vi "Set BUZZ.vi"(10 "Inetensity":dbl, 11 "BUZZ Select":T1) -> (3 "Controller BUZZ":T2)   [LabVIEW 2020, in "GameController_SEN.lvlib"]
uses:
  GameController_SEN.lvlib
  Shared Code/TypeDefs/Cluster_Controller Buzz.ctl
  Shared Code/TypeDefs/ENUM_Controller Buzz Select.ctl
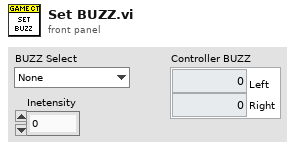
[diagram p1: front panel]
types:
  T1 = typedef "ENUM_Controller Buzz Select.ctl" = enum16{"None", "Timed Full ON", "Set Intensity", ".5 Sec Cycle Count"}
  T2 = typedef "Cluster_Controller Buzz.ctl" = cluster{"Left":dbl, "Right":dbl}
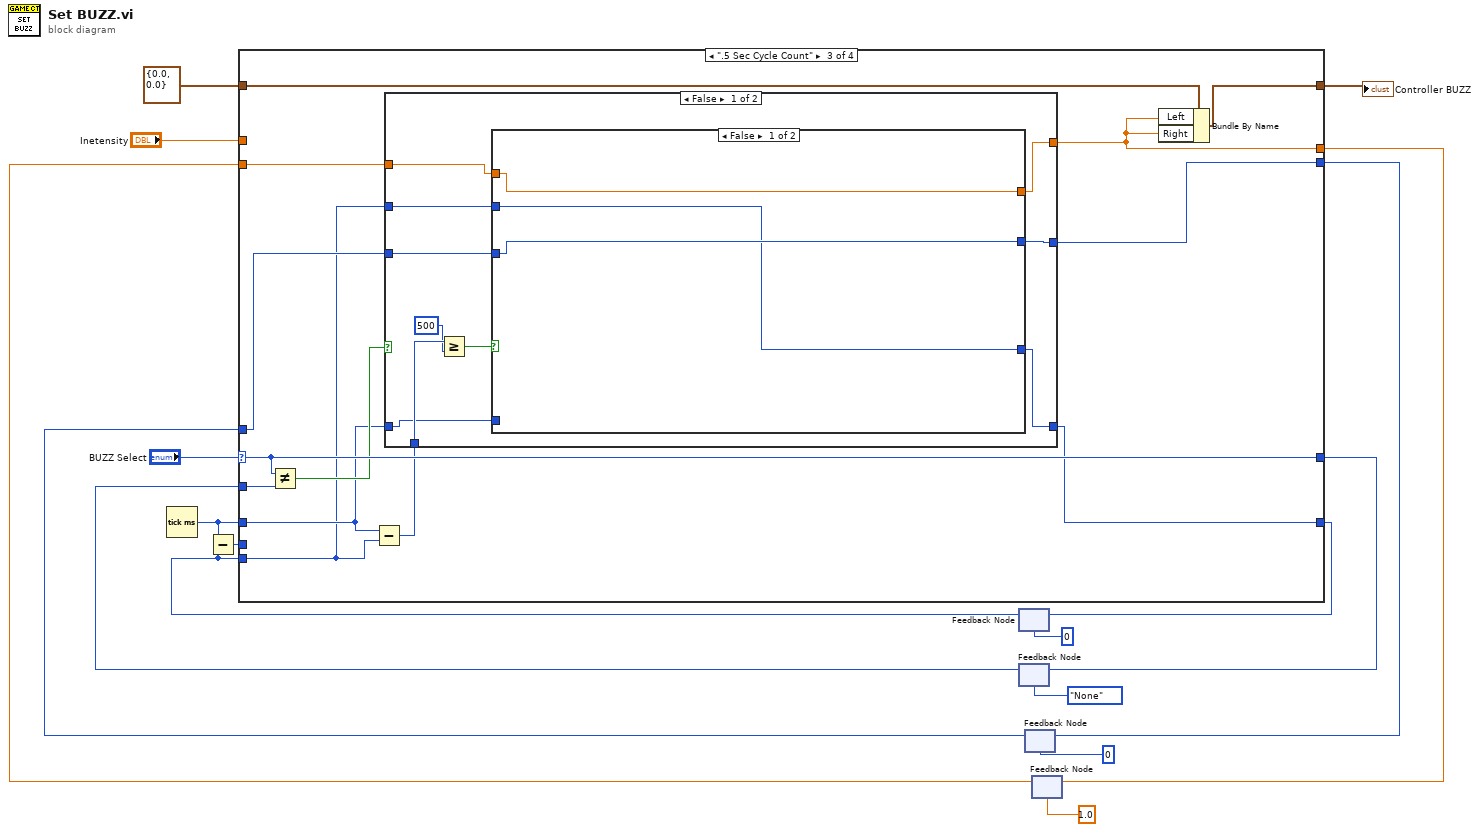
[diagram p0: block diagram]
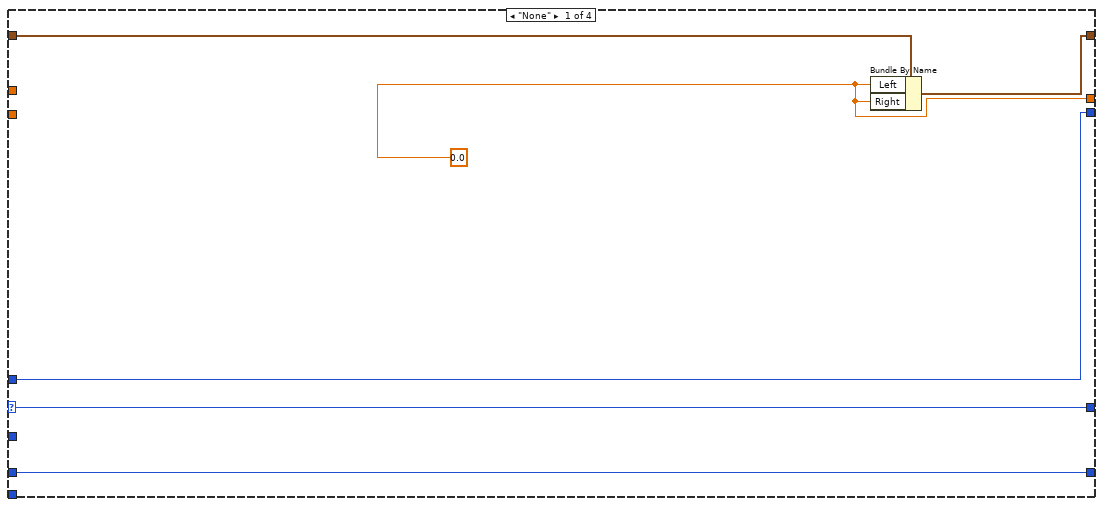
[diagram p2: hidden frame]
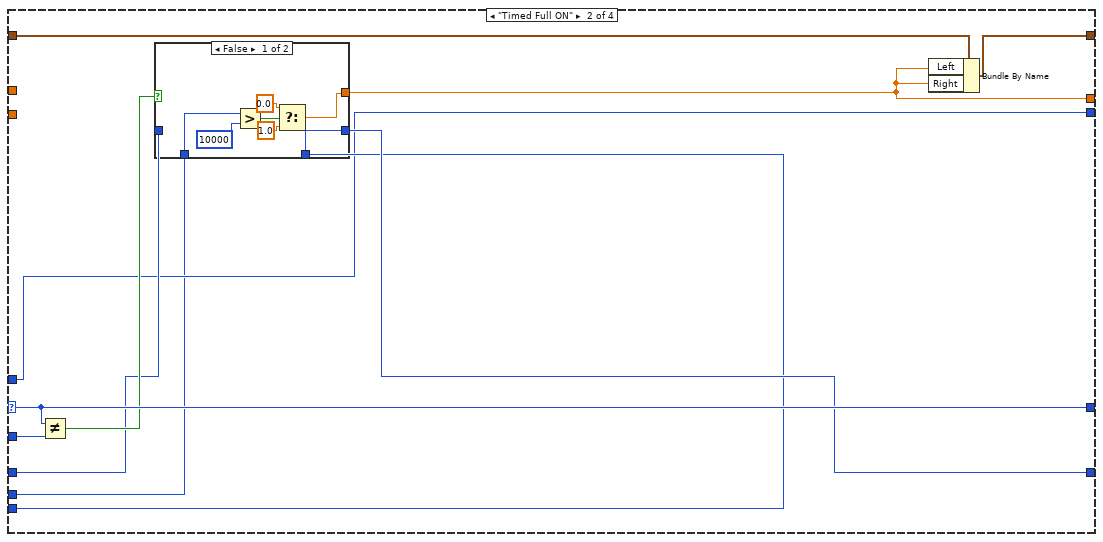
[diagram p3: hidden frame]
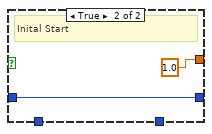
[diagram p4: hidden frame]
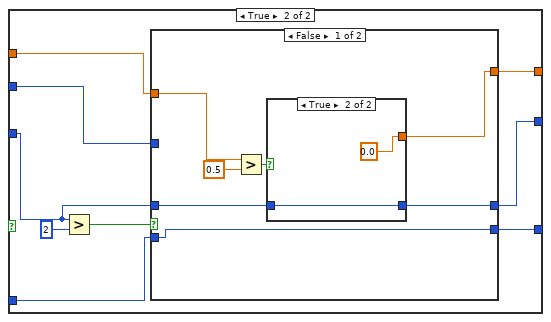
[diagram p5: hidden frame]
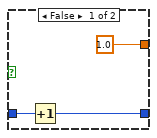
[diagram p6: hidden frame]
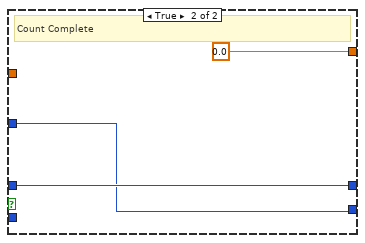
[diagram p7: hidden frame]
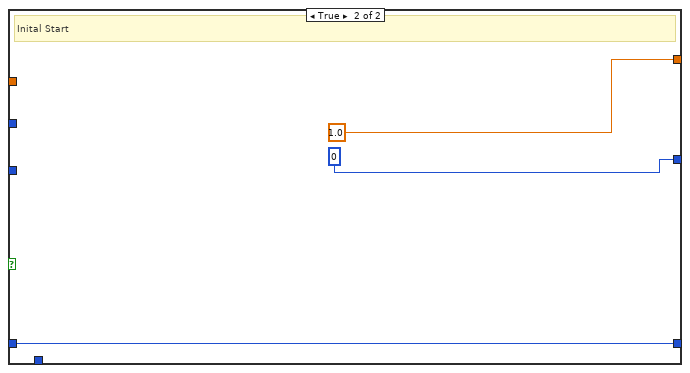
[diagram p8: hidden frame]
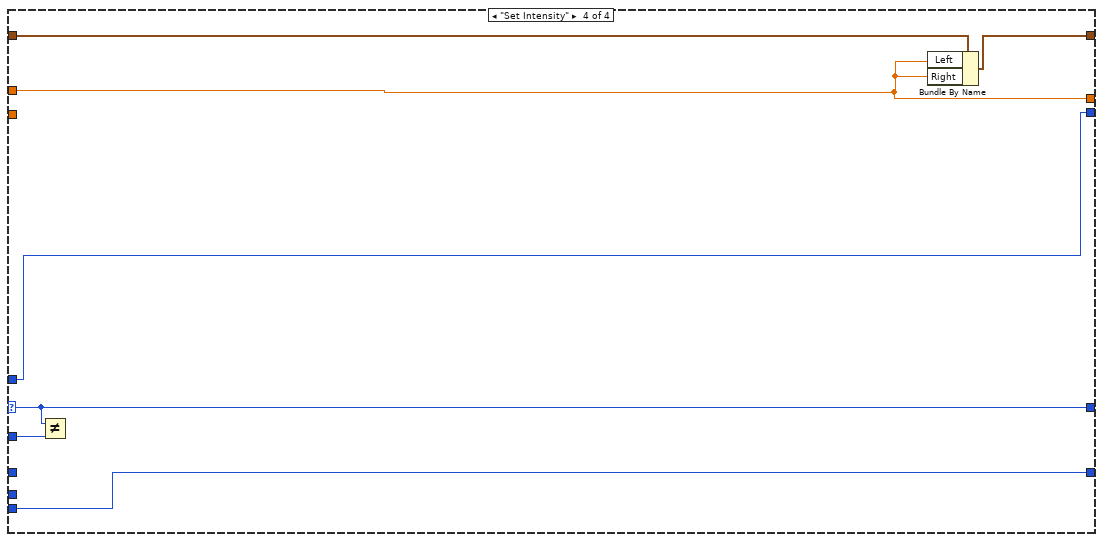
[diagram p9: hidden frame]
diagram:
  n1 = Tick Count (ms)() -> (millisecond timer value=w3:u32)
  n2 = feedback #1(u32 0 ("millisecond timer value")) -> (w2:u32)
  n3 = Subtract(x=w3, y=w2) -> (x-y=w1:u32)
  n4 = feedback #2(ENUM_Controller_Buzz_Select."None" ("BUZZ Select")) -> (w12:T1)
  n5 = feedback #3(0) -> (w8:i32)
  n6 = feedback #4(1.0) -> (w5:dbl)
  n7 = case shown="\".5 Sec Cycle Count\"" "BUZZ Select" {
    selector: "BUZZ Select" -> [w21 w33 w55 w102]
    tunnel: T2 {"Left"=0.0, "Right"=0.0} ("Controller BUZZ") -> [w24 w35 w57 w104]
    tunnel: [w23 w34 w56 w103] -> w16
    tunnel: w3 -> [w22 w29 w51 _]
    tunnel: [w22 w30 w52 w98] -> w15
    tunnel: w2 -> [_ w28 w45 w98]
    tunnel: [w21 w33 w55 w102] -> w13
    tunnel: w12 -> [_ w32 w54 w101]
    tunnel: [w19 w27 w49 w100] -> w10
    tunnel: w8 -> [w19 w27 w48 w100]
    tunnel: [w20 w26 w47 w99] -> w7
    tunnel: w5 -> [_ _ w46 _]
    tunnel: "Inetensity" -> [_ _ _ w99]
    tunnel: w1 -> [_ w25 _ _]
    frame "None" {
      w20 = 0.0 ("Left")
      n8 = Bundle By Name(cluster=w24, "Left"=w20, "Right"=w20) -> (w23:T2)
    }
    frame "Timed Full ON" {
      n9 = Not Equal?(x=w33, y=w32) -> (x != y?=w31:bool)
      n10 = case shown="False" w31 {
        tunnel: [w38 1.0] -> w26
        tunnel: w29 -> [_ w43]
        tunnel: [w42 w43] -> w30
        tunnel: w28 -> [w42 _]
        tunnel: w25 -> [w41 _]
        frame False {
          n11 = Greater?(x=w41, y=u32 10000) -> (0:w39:bool)
          n12 = Select(t=0.0, s=w39, f=1.0) -> (s? t:f=w38:dbl)
        }
        frame True {
          # "Inital Start"
        }
      }
      n13 = Bundle By Name(cluster=w35, "Left"=w26, "Right"=w26) -> (w34:T2)
    }
    frame ".5 Sec Cycle Count" {
      n14 = Not Equal?(x=w55, y=w54) -> (x != y?=w53:bool)
      n15 = Subtract(x=w51, y=w45) -> (x-y=w50:u32)
      n16 = case shown="False" w53 {
        tunnel: [w62 1.0] -> w47
        tunnel: w51 -> [w58 w96]
        tunnel: [w59 w96] -> w52
        tunnel: w50 -> [w67 _]
        tunnel: [w61 0] -> w49
        tunnel: w48 -> [w63 _]
        tunnel: w46 -> [w64 _]
        tunnel: w45 -> [w60 _]
        frame False {
          n17 = Greater Or Equal?(x=w67, y=u32 500) -> (x >= y?=w65:bool)
          n18 = case shown="False" w65 {
            tunnel: w64 -> [w70 w71]
            tunnel: w63 -> [w69 w75]
            tunnel: [w70 w77] -> w62
            tunnel: [w69 w76] -> w61
            tunnel: w60 -> [w68 w74]
            tunnel: [w68 w73] -> w59
            tunnel: w58 -> [_ w72]
            frame False {
            }
            frame True {
              n19 = Greater?(x=w75, y=2) -> (0:w78:bool)
              n20 = case shown="False" w78 {
                tunnel: [w80 0.0] -> w77
                tunnel: [w85 w93] -> w76
                tunnel: w75 -> [w86 w93]
                tunnel: [w84 w92] -> w73
                tunnel: w74 -> [_ w92]
                tunnel: w72 -> [w84 _]
                tunnel: w71 -> [w83 _]
                frame False {
                  n21 = Greater?(x=w83, y=0.5) -> (0:w81:bool)
                  n22 = case shown="True" w81 {
                    tunnel: w86 -> [w89 w91]
                    tunnel: [w88 w91] -> w85
                    tunnel: [1.0 0.0] -> w80
                    frame False {
                      n23 = Increment(x=w89) -> (x+1=w88:i32)
                    }
                    frame True {
                    }
                  }
                }
                frame True {
                  # "Count Complete"
                }
              }
            }
          }
        }
        frame True {
          # "Inital Start"
        }
      }
      n24 = Bundle By Name(cluster=w57, "Left"=w47, "Right"=w47) -> (w56:T2)
    }
    frame "Set Intensity" {
      n25 = Not Equal?(x=w102, y=w101) -> ()  [unwired: 1 out]
      n26 = Bundle By Name(cluster=w104, "Left"=w99, "Right"=w99) -> (w103:T2)
    }
  }
  "Controller BUZZ" <- w16
  n27 = feedback-in #1(w15) -> ()
  n28 = feedback-in #2(w13) -> ()
  n29 = feedback-in #3(w10) -> ()
  n30 = feedback-in #4(w7) -> ()
